vi "Spy Dequeue Call.vi"(8 "error in (no error)":errorcluster, 9 "timeout in ms (-1)":i32, 11 "Mock Process In":refnum<class "Mock Process.lvclass">) -> (0 "error out":errorcluster, 1 "Message Data":variant, 2 "Message":string, 3 "Mock Process Out":refnum<class "Mock Process.lvclass">, 4 "timed out?":bool)   [LabVIEW 2020, in "Mock Process.lvclass"]
doc: "Spys on errors sent to the error handler. This Method requires a lock on the execution thread to prevent race conditions when testing other processes using the error handler."
uses:
  Mock Process.lvclass
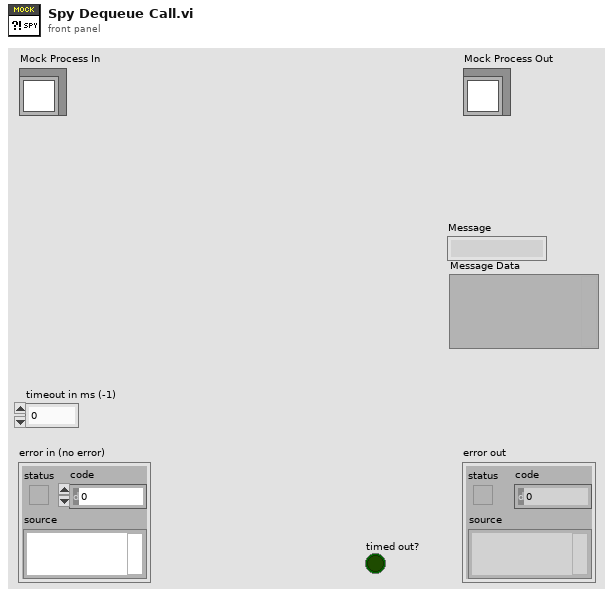
[diagram p1: front panel]
types:
  T1 = cluster{"Message":string, "Message Data":variant}
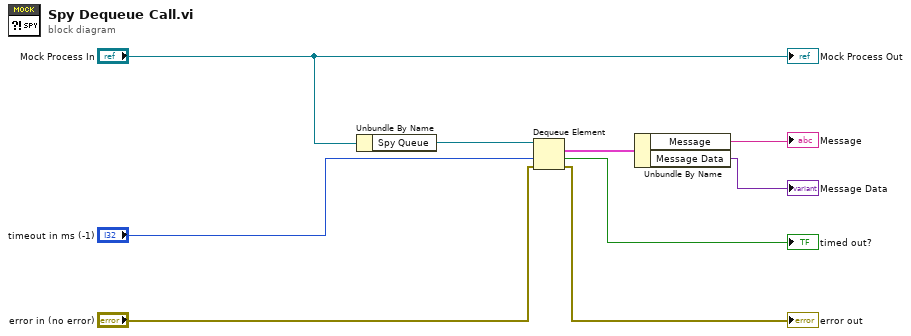
[diagram p0: block diagram]
diagram:
  n1 = Unbundle By Name("Mock Process In") -> ("Spy Queue"=w8:refnum<queue>)
  n2 = Dequeue Element(queue=w8, timeout in ms (-1)="timeout in ms (-1)", error in (no error)="error in (no error)") -> (element=w3:T1, timed out?=→"timed out?":bool, error out=→"error out":errorcluster)  [unwired: 1 out]
  n3 = Unbundle By Name(w3) -> ("Message"=→"Message":string, "Message Data"=→"Message Data":variant)
  "Mock Process Out" <- "Mock Process In"
